vi "hpanel_message_panel.vi"(8 "error in (no error)":errorcluster, 10 "event data":T1, 11 "hydraharp_panel in":refnum<class "hydraharp_panel.lvclass">) -> (0 "error out":errorcluster, 3 "hydraharp_panel out":refnum<class "hydraharp_panel.lvclass">)   [LabVIEW 2015, in "hydraharp_panel.lvclass"]
uses:
  hydraharp_panel.lvclass
  hpanel_messages_to_panel_from_actor_loop.ctl
  hydraharp_panel.lvclass/hydraharp_panel.ctl
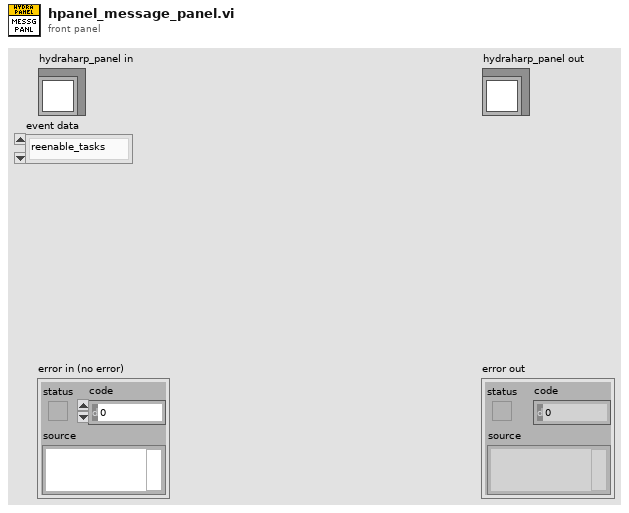
[diagram p1: front panel]
types:
  T1 = typedef "hpanel_messages_to_panel_from_actor_loop.ctl" = enum16{"reenable_tasks"}
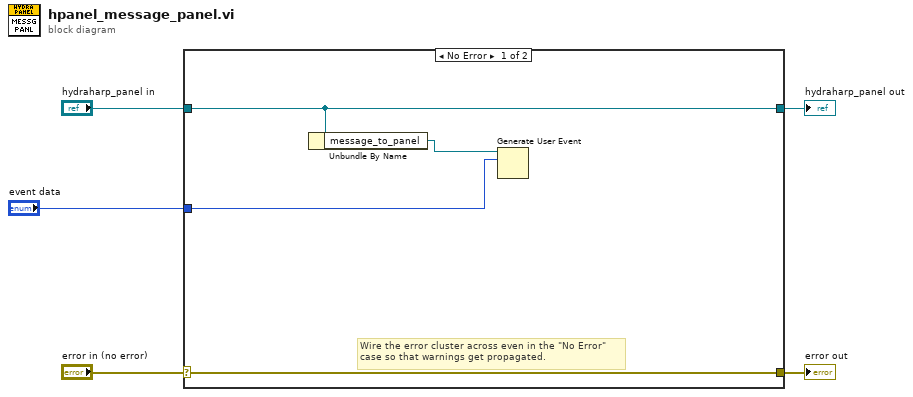
[diagram p0: block diagram]
diagram:
  n1 = case shown="No Error" "error in (no error)" {
    selector: "error in (no error)" -> [w9 w11]
    tunnel: [w9 w11] -> w4
    tunnel: [w8 w10] -> w2
    tunnel: "hydraharp_panel in" -> [w8 w10]
    tunnel: "event data" -> [w6 _]
    frame No Error {
      # "Wire the error cluster across even in the \"No Error\"\ncase so that warnings get propagated."
      n2 = Unbundle By Name(w8) -> ("message_to_panel"=w7:refnum<user-event>)
      n3 = Generate User Event(user event=w7, event data cluster=w6) -> ()  [unwired: 2 in, 2 out]
    }
    frame Error {
    }
  }
  "error out" <- w4
  "hydraharp_panel out" <- w2
